vi "SequenceIndicesTCMouseDown.vi"(8 "error in (no error)":errorcluster, 10 "MouseDownIn":T2, 11 "VMUI in":refnum<class "VMUI.lvclass">) -> (0 "error out":errorcluster, 2 "MouseDownOut":T3, 3 "VMUI out":refnum<class "VMUI.lvclass">)   [LabVIEW 2013, in "VMUI.lvclass"]
uses:
  VMUI.lvclass
  <vilib>/Utility/miscctls.llb/LVPoint32TypeDef.ctl
  <vilib>/Utility/miscctls.llb/LVRowAndColumnTypeDef.ctl
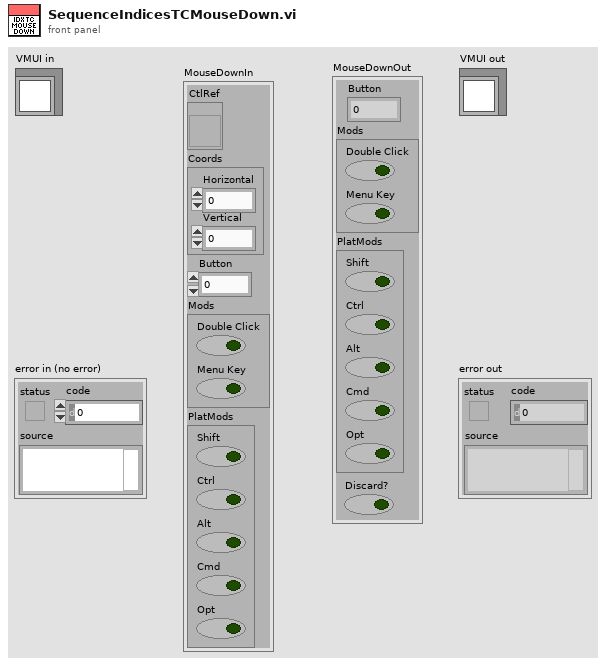
[diagram p1: front panel]
types:
  T1 = typedef "LVPoint32TypeDef.ctl" = cluster{"Horizontal":i32, "Vertical":i32}
  T2 = cluster{"CtlRef":refnum<vi>, "Coords":T1, "Button":u16, "Mods":cluster{"Double Click":bool, "Menu Key":bool}, "PlatMods":cluster{"Shift":bool, "Ctrl":bool, "Alt":bool, "Cmd":bool, "Opt":bool}}
  T3 = cluster{"Button":u16, "Mods":cluster{"Double Click":bool, "Menu Key":bool}, "PlatMods":cluster{"Shift":bool, "Ctrl":bool, "Alt":bool, "Cmd":bool, "Opt":bool}, "Discard?":bool}
  T4 = typedef "LVRowAndColumnTypeDef.ctl" = cluster{"Row":i32, "Column":i32}
  T5 = cluster{"Shift":bool, "Ctrl":bool, "Alt":bool, "Cmd":bool, "Opt":bool}
  T6 = cluster{"Button":u16, "Mods":cluster{"Double Click":bool, "Menu Key":bool}, "PlatMods":cluster{"Shift":bool, "Ctrl":bool, "Alt":bool, "Cmd":bool, "Opt":bool}, bool}
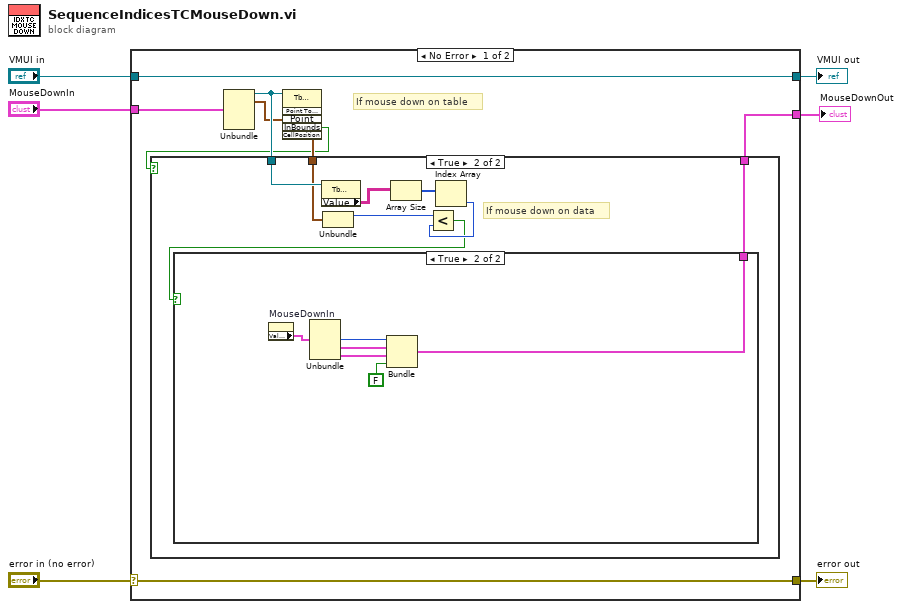
[diagram p0: block diagram]
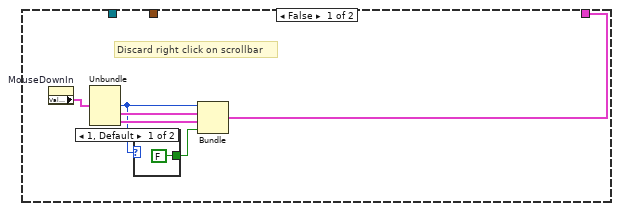
[diagram p2: hidden frame]
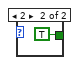
[diagram p3: hidden frame]
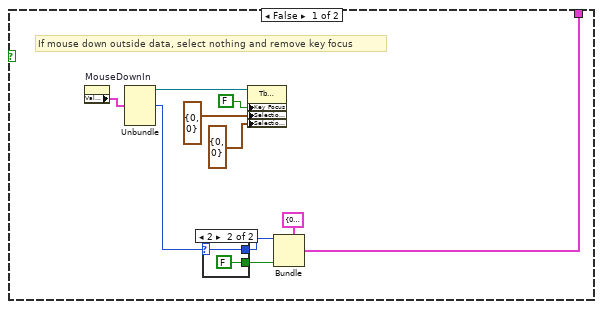
[diagram p4: hidden frame]
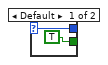
[diagram p5: hidden frame]
diagram:
  n1 = case shown="No Error" "error in (no error)" {
    selector: "error in (no error)" -> [w13 w52]
    tunnel: [w13 w52] -> w5
    tunnel: [w14 w51] -> w3
    tunnel: "VMUI in" -> [w14 w51]
    tunnel: [w8 _] -> w2
    tunnel: "MouseDownIn" -> [w7 _]
    frame No Error {
      # "If mouse down on table"
      n2 = Unbundle(w7) -> ("CtlRef"=w12:refnum<vi>, "Coords"=w9:T1)  [unwired: 3 out]
      n3 = invoke class="Tbl (strict)" method="Point To Row Column"(reference=w12, "Point"=w9) -> ("InBounds"=w10:bool, "CellPosition"=w11:T4)  [unwired: 4 in, 4 out]
      n4 = case shown="True" w10 {
        tunnel: [w19 w26] -> w8
        tunnel: w11 -> [_ w24]
        tunnel: w12 -> [_ w25]
        frame False {
          # "Discard right click on scrollbar"
          n5 = property on="MouseDownIn" class="Clust (strict)"() -> ("Value"=w18:T2)  [unwired: 2 in, 2 out]
          n6 = Unbundle(w18) -> ("Button"=w15:u16, "Mods"=w17:cluster{"Double Click":bool, "Menu Key":bool}, "PlatMods"=w16:T5)  [unwired: 2 out]
          n7 = case shown="1, Default" w15 {
            tunnel: [FALSE TRUE] -> w20
            frame 1, Default {
            }
            frame 2 {
            }
          }
          n8 = Bundle("Button"=w15, "Mods"=w17, "PlatMods"=w16, w20) -> (w19:T6)  [unwired: 1 in]
        }
        frame True {
          # "If mouse down on data"
          n9 = property class="Tbl (strict)"(reference=w25) -> ("Value"=w30:string[][])  [unwired: 1 in, 2 out]
          n10 = Unbundle(w24) -> ("Row"=w27:i32)  [unwired: 1 out]
          n11 = Array Size(array=w30) -> (size(s)=w29:i32[])
          n12 = Index Array(array=w29) -> (element=w28:i32)  [unwired: 1 in]
          n13 = Less?(x=w27, y=w28) -> (x < y?=w23:bool)
          n14 = case shown="True" w23 {
            tunnel: [w31 w45] -> w26
            frame False {
              # "If mouse down outside data, select nothing and remove key focus"
              n15 = property on="MouseDownIn" class="Clust (strict)"() -> ("Value"=w32:T2)  [unwired: 2 in, 2 out]
              n16 = Unbundle(w32) -> ("CtlRef"=w33:refnum<vi>, "Button"=w37:u16)  [unwired: 3 out]
              n17 = case shown="2" w37 {
                selector: w37 -> [w42 w43]
                tunnel: [TRUE FALSE] -> w38
                tunnel: [w42 w43] -> w39
                frame Default {
                }
                frame 2 {
                }
              }
              n18 = property class="Tbl (strict)"(reference=w33, "Key Focus"=FALSE, "Selection Size"=T4 {"Row"=0, "Column"=0}, "Selection Start"=T4 {"Row"=0, "Column"=0}) -> ()  [unwired: 1 in, 2 out]
              n19 = Bundle(cluster=T3 {"Button"=0, "Mods"={"Double Click"=FALSE, "Menu Key"=FALSE}, "PlatMods"={"Shift"=FALSE, "Ctrl"=FALSE, "Alt"=FALSE, "Cmd"=FALSE, "Opt"=FALSE}, "Discard?"=TRUE} ("MouseDownOut"), "Button"=w39, "Discard?"=w38) -> (w31:T3)  [unwired: 2 in]
            }
            frame True {
              n20 = property on="MouseDownIn" class="Clust (strict)"() -> ("Value"=w49:T2)  [unwired: 2 in, 2 out]
              n21 = Unbundle(w49) -> ("Button"=w46:u16, "Mods"=w48:cluster{"Double Click":bool, "Menu Key":bool}, "PlatMods"=w47:T5)  [unwired: 2 out]
              n22 = Bundle("Button"=w46, "Mods"=w48, "PlatMods"=w47, FALSE) -> (w45:T6)  [unwired: 1 in]
            }
          }
        }
      }
    }
    frame Error {
    }
  }
  "error out" <- w5
  "VMUI out" <- w3
  "MouseDownOut" <- w2
